vi "HMI.vi"(8 "error in (no error)":errorcluster caption="entrée d'erreur (pas d'erreur)", 11 "Class Popup Operator_Validation (Default) en entrée":refnum<class "Class Popup Result_Info (Virtual).lvclass">) -> (0 "error out":errorcluster caption="sortie d'erreur", 1 "Input":string, 2 "Operator_Selection":bool, 3 "Class Popup Operator_Validation (Default) en sortie":refnum<class "Class Popup Result_Info (Virtual).lvclass">)   [LabVIEW 2020, in "Library Instrument & Equipement.lvlib" / "Library Popup.lvlib" / "Class Popup Result_Info (Virtual).lvclass"]
uses:
  Class Popup Result_Info (Virtual).lvclass
  Class Popup (Main)/Class Popup (Main).lvclass
panel:
  in  "Bouton OK":bool caption="Validated"
  in  "Arbre Liste SN":string[](tree)
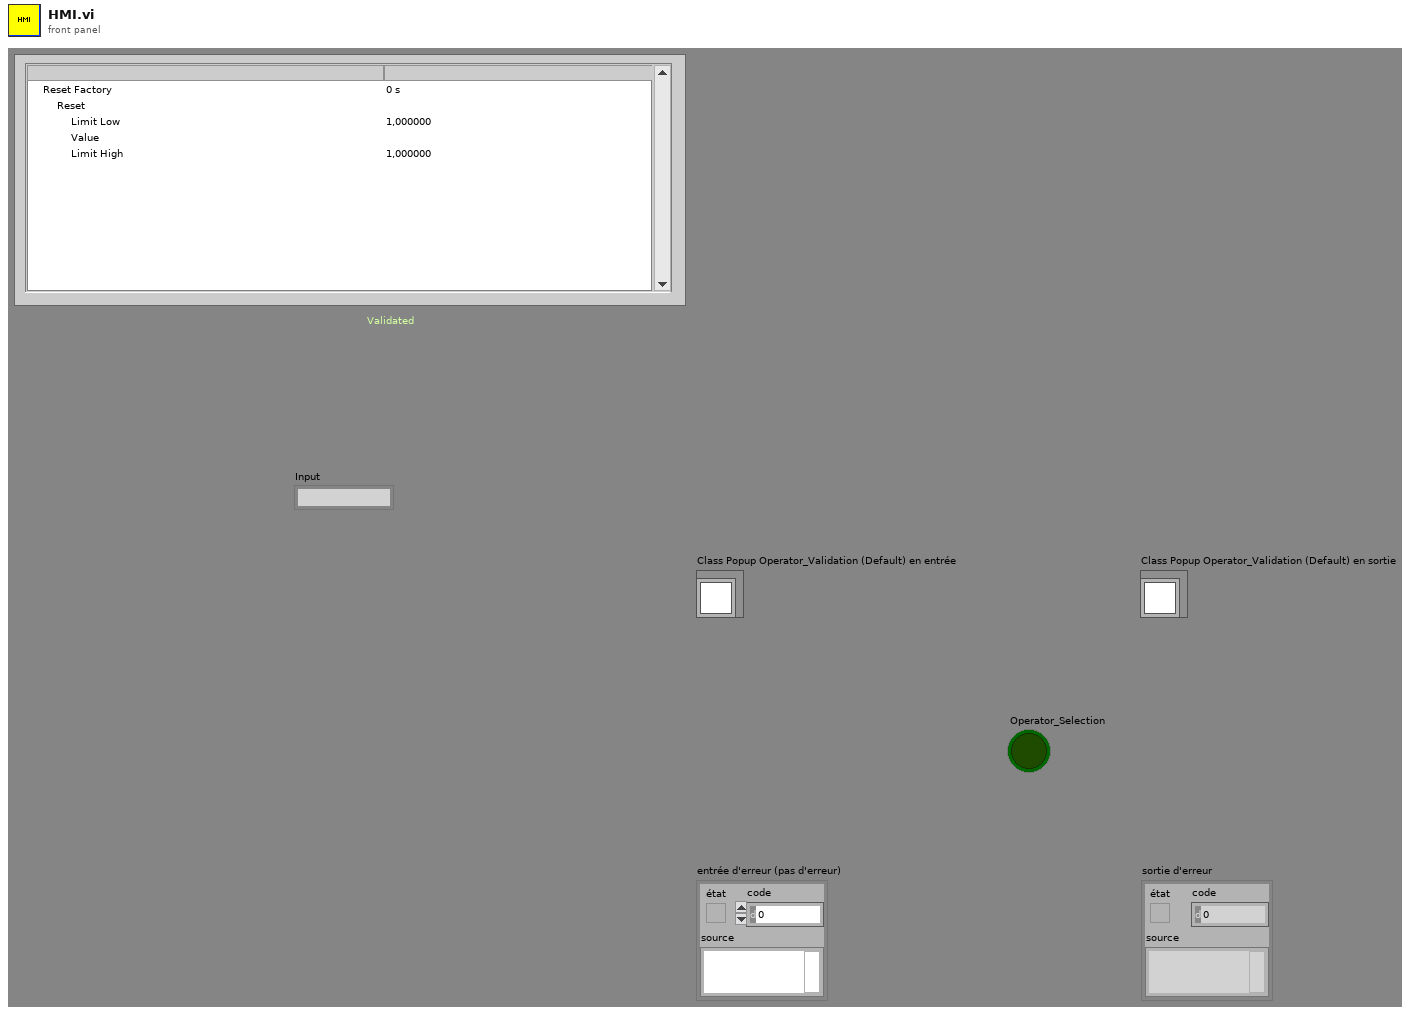
[diagram p1: front panel]
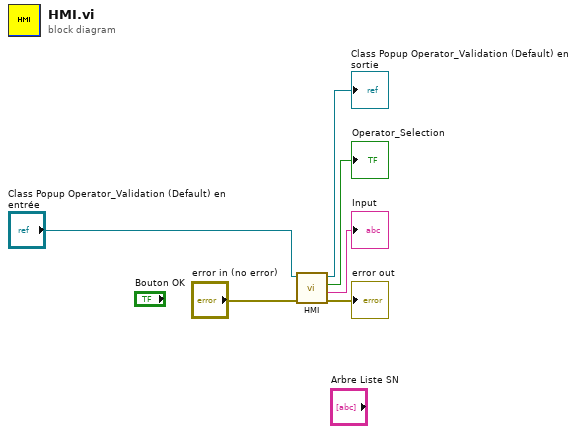
[diagram p0: block diagram]
diagram:
  n1 = call-parent "HMI.vi"("error in (no error)"="error in (no error)", "Class Popup (Main) en entrée"="Class Popup Operator_Validation (Default) en entrée") -> ("error out"=→"error out":errorcluster, "Input"=→"Input":string, "Operator_Selection"=→"Operator_Selection":bool, "Class Popup (Main) en sortie"=→"Class Popup Operator_Validation (Default) en sortie":refnum<class "Class Popup Result_Info (Virtual).lvclass">)  [unwired: 6 in]
